vi "Test Binary Serialisation.vi"() -> ()   [LabVIEW 2021]
uses:
  Source/Variables/Support/Bool/Var_Bool.lvclass
  C:/New folder/LV_Abstract/LV_Abstract/Source/Abs_Types/Boolean/Abs_Boolean.lvclass
  Source/Variables/Support/Bool/Support/Init_Simple_Var.vi
  Source/Abs_Types/Boolean/Simple Read.vi
  Source/Abs_Types/Boolean/Abs_Boolean.lvclass
  Source/Constants/Support/Bool/Bool.vi
  Source/Constants/Support/Bool/Const_Bool.lvclass
  Source/Constants/Support/DBL/DBL.vi
  Source/Constants/Support/DBL/Const_DBL.lvclass
  Source/Abs_Types/Type/Abs_Type.lvclass
  Source/Abs_Types/Double Float/Simple Read.vi
  Source/Abs_Types/Double Float/Abs_Double Float.lvclass
  Source/Functions/Logic/Support/OR/Bool/Method.vi
  Source/Functions/Logic/Support/OR/Bool/OR_Bool.lvclass
  C:/New folder/LV_Abstract/LV_Abstract/Source/Abs_Types/Value/Abs_Value.lvclass
  C:/New folder/LV_Abstract/LV_Abstract/Source/Abs_Types/Type/Abs_Type.lvclass
  C:/New folder/LV_Abstract/LV_Abstract/Source/Variables/Support/Bool/Var_Bool.lvclass
panel:
  in  "Value":bool
  in  "Boolean 5":bool
  out "Binary 4":string
  out "Boolean 4":bool
  in  "Boolean 3":bool
  out "Numeric 2":dbl
  in  "Numeric":dbl
  out "Binary 3":string
  out "Boolean":bool
  out "Binary 2":string
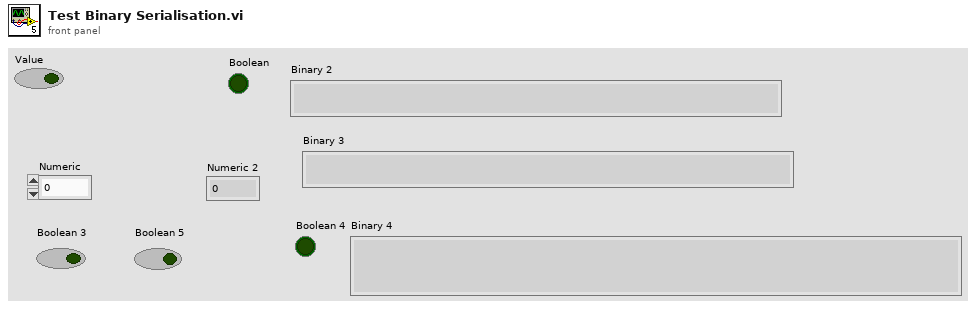
[diagram p1: front panel]
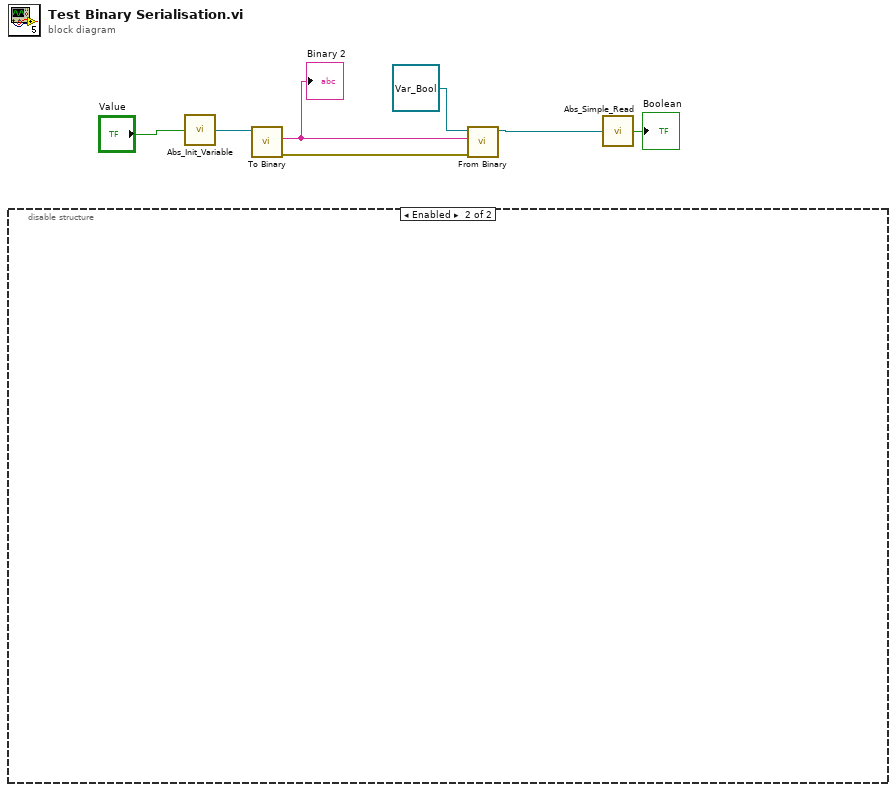
[diagram p0: block diagram]
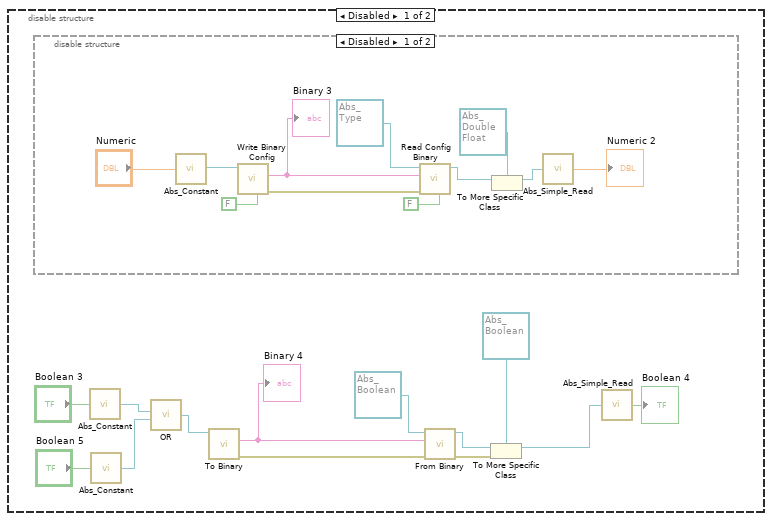
[diagram p2: hidden frame]
diagram:
  n1 = disable-structure shown="Enabled" {
    frame Disabled {
      n2 = disable-structure shown="Disabled" {
        frame Disabled {
          n3 = call-poly "Abs_Constant.vi"("Value"="Numeric") -> ("Constant"=w31:refnum<class "Const_DBL.lvclass">)  [unwired: 4 in]
          n4 = call-dynamic "Write Binary Config.vi"("Include Class Name"=FALSE, "Const_DBL in"=w31) -> ("error out"=w25:errorcluster, "Binary"=w24:string)  [unwired: 7 in, 1 out]
          "Binary 3" <- w24
          n5 = call "Read Config Binary.vi"("Class Name is Included"=FALSE, "error in (no error)"=w25, "Binary"=w24, "Abs_Type in"=refnum<class "Abs_Type.lvclass"> refnum ("Abs_Type.lvclass")) -> ("Abs_Type out"=w21:refnum<class "Abs_Type.lvclass">)  [unwired: 5 in, 2 out]
          n6 = To More Specific Class(target class=refnum<class "Abs_Double Float.lvclass"> refnum ("Class"), reference=w21) -> (specific class reference=w27:refnum<class "Abs_Double Float.lvclass">)  [unwired: 1 in, 1 out]
          n7 = call-poly "Abs_Simple_Read.vi"("Class"=w27) -> ("Value"=→"Numeric 2":dbl)  [unwired: 4 in]
        }
        frame Enabled {
        }
      }
      n8 = call-poly "Abs_Constant.vi"("Boolean"="Boolean 3") -> ("Abs_Boolean.lvclass"=w13:refnum<class "Abs_Boolean.lvclass">)  [unwired: 4 in]
      n9 = call-poly "Abs_Constant.vi"("Boolean"="Boolean 5") -> ("Abs_Boolean.lvclass"=w11:refnum<class "Abs_Boolean.lvclass">)  [unwired: 4 in]
      n10 = call-poly "OR.vi"("B"=w11, "A"=w13) -> ("Result"=w10:refnum<class "Abs_Boolean.lvclass">)  [unwired: 4 in]
      n11 = call-dynamic "To Binary.vi"("Boolean in"=w10) -> ("error out"=w20:errorcluster, "Binary"=w19:string)  [unwired: 8 in, 1 out]
      "Binary 4" <- w19
      n12 = call-dynamic "From Binary.vi"("error in (no error)"=w20, "Binary"=w19, "Boolean in"=refnum<class "Abs_Boolean.lvclass"> refnum) -> ("error out"=w17:errorcluster, "Boolean out"=w18:refnum<class "Abs_Boolean.lvclass">)  [unwired: 6 in, 1 out]
      n13 = To More Specific Class(target class=refnum<class "Abs_Boolean.lvclass"> refnum ("Abs_Boolean.lvclass"), reference=w18, error in=w17) -> (specific class reference=w9:refnum<class "Abs_Boolean.lvclass">)  [unwired: 1 out]
      n14 = call-poly "Abs_Simple_Read.vi"("Boolean in"=w9) -> ("Boolean"=→"Boolean 4":bool)  [unwired: 4 in]
    }
    frame Enabled {
    }
  }
  n15 = call-poly "Abs_Init_Variable.vi"("Value"="Value") -> ("Var"=w2:refnum<class "Var_Bool.lvclass">)  [unwired: 4 in]
  n16 = call-dynamic "To Binary.vi"("Boolean in"=w2) -> ("error out"=w5:errorcluster, "Binary"=w6:string)  [unwired: 8 in, 1 out]
  "Binary 2" <- w6
  n17 = call-dynamic "From Binary.vi"("error in (no error)"=w5, "Binary"=w6, "Boolean in"=refnum<class "Var_Bool.lvclass"> refnum ("Var_Bool.lvclass")) -> ("Boolean out"=w4:refnum<class "Var_Bool.lvclass">)  [unwired: 6 in, 2 out]
  n18 = call-poly "Abs_Simple_Read.vi"("Boolean in"=w4) -> ("Boolean"=→"Boolean":bool)  [unwired: 4 in]
